vi "Test Get Item by ID.vi"(8 "error in (no error)":errorcluster, 11 "Test Case In":refnum<class "Debugger Test.lvclass">) -> (0 "error out":errorcluster, 3 "Test Case Out":refnum<class "Debugger Test.lvclass">)   [LabVIEW 2020, in "Debugger Test.lvclass"]
uses:
  Debugger Test.lvclass
  C:/Program Files (x86)/National Instruments/LabVIEW 2020/vi.lib/Astemes/LUnit/Test Case.lvclass
  source/Debugger/Debugger.lvclass
  C:/Users/anton/Documents/GitHub/triarc-debugger/source/Process/Debug Process.lvclass
  source/Debug Data/Raw Debug Data.ctl
  source/Debug Data/Debug Data.lvclass/Debug Data.ctl
  source/Process/Debug Process.lvclass/Debug Process.ctl
  <vilib>/Astemes/LUnit/Test Case.lvclass/Test Case.ctl
  <vilib>/Astemes/LUnit/LUnit Assertion Result.lvclass/LUnit Assertion Result.ctl
  <vilib>/Astemes/LUnit/LUnit Test Case Result.lvclass/LUnit Test Case Result.ctl
  <vilib>/Astemes/LUnit/LUnit Method Result.lvclass/LUnit Method Result.ctl
  01074fa8-ee8a-411d-bc8b-fc92c4f90959.vi
  source/Process/Private/SubVIs/Wait for finish.vi
  source/Process/Protected/Messaging/Enqueue Message.vi
  source/Process/Private/SubVIs/Set Lifecycle State.vi
  source/Process/Public/Lifecycle/Get Lifecycle State.vi
  <vilib>/Astemes/LUnit/Palette/Pass.vi
  <vilib>/Astemes/LUnit/Palette/Fail.vi
  <vilib>/Astemes/LUnit/Compare Variants.vi
  <vilib>/Astemes/LUnit/Describe Comparison.vi
  <vilib>/Astemes/LUnit/Set Assertion Type.vi
  <vilib>/Utility/error.llb/Clear Errors.vi
  <vilib>/Astemes/LUnit/Add test result.vi
  <vilib>/Astemes/LUnit/LUnit Write Passed.vi
  <vilib>/Astemes/LUnit/LUnit Write Message.vi
  <vilib>/Astemes/LUnit/LUnit Write Description.vi
  <vilib>/Astemes/LUnit/Variant to string.vi
  <vilib>/Astemes/LUnit/LUnit Write Assertion Type.vi
  <vilib>/Astemes/LUnit/LUnit Record Assertion Result.vi
  <vilib>/Astemes/LUnit/LUnit Aggregate Assertion Results.vi
  <vilib>/Astemes/LUnit/Assertion Result/LUnit Read Status.vi
  <vilib>/Astemes/LUnit/LUnit Read Message.vi
  <vilib>/Astemes/LUnit/LUnit Read Description.vi
  <vilib>/Astemes/LUnit/Method Result/LUnit Merge Status.vi
  <vilib>/Astemes/LUnit/LUnit Concatenate result strings.vi
  <vilib>/Utility/error.llb/Error Cluster From Error Code.vi
  <vilib>/Utility/Data Type/Get Type Information.vi
  <vilib>/Utility/LVClass/Get LV Class Name.vi
  <vilib>/Astemes/LUnit/LUnit Assertion Result.lvclass
  source/Process/Debug Process.lvclass
  source/Debug Data/Debug Data.lvclass
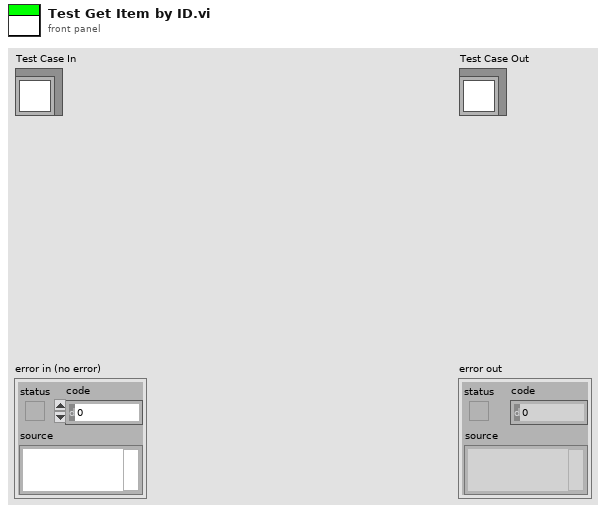
[diagram p1: front panel]
types:
  T1 = typedef "Debug Data.lvclass/Raw Debug Data.ctl" = cluster{"Action":string, "Call Chain":string, "Process":string, "Message":string, "Message Data":variant, "Time":dbl}
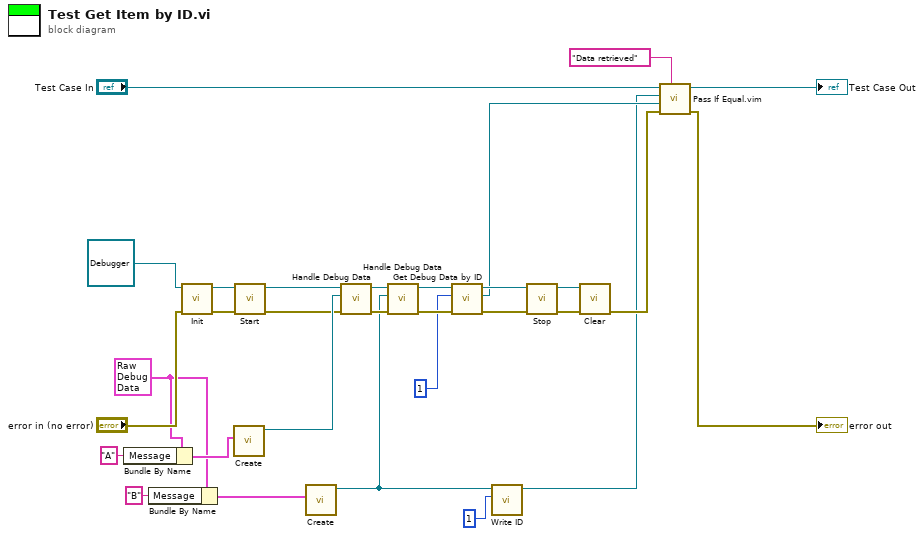
[diagram p0: block diagram]
diagram:
  w11 = T1 {"Action"="", "Call Chain"="", "Process"="", "Message"="", "Message Data"=variant, "Time"=0.0} ("Debug Data Cluster")
  n1 = Bundle By Name(cluster=w11, "Message"="A" ("Process")) -> (w18:T1)
  n2 = Bundle By Name(cluster=w11, "Message"="B" ("Process")) -> (w12:T1)
  n3 = call-dynamic "Init.vi"("error in (no error)"="error in (no error)", "Process In"=refnum<class "Debugger.lvclass"> refnum ("Debug Data Event In 2")) -> ("error out"=w26:errorcluster, "Process Out"=w27:refnum<class "Debugger.lvclass">)  [unwired: 8 in]
  n4 = call "Create.vi"("Debug Data Cluster"=w18) -> ("Debug Data out"=w19:refnum<class "Debug Data.lvclass">)  [unwired: 9 in, 1 out]
  n5 = call "Start.vi"("error in (no error)"=w26, "Process In"=w27) -> ("error out"=w4:errorcluster, "Process Out"=w5:refnum<class "Debugger.lvclass">)  [unwired: 7 in, 1 out]
  n6 = call "Create.vi"("Debug Data Cluster"=w12) -> ("Debug Data out"=w6:refnum<class "Debug Data.lvclass">)  [unwired: 9 in, 1 out]
  n7 = call-dynamic "Handle Debug Data.vi"("error in (no error)"=w4, "Debug Data.lvclass"=w19, "Debug Data Event In"=w5) -> ("error out"=w15:errorcluster, "Debug Data Event Out"=w16:refnum<class "Debugger.lvclass">)  [unwired: 7 in]
  n8 = call-dynamic "Handle Debug Data.vi"("error in (no error)"=w15, "Debug Data.lvclass"=w6, "Debug Data Event In"=w16) -> ("error out"=w14:errorcluster, "Debug Data Event Out"=w9:refnum<class "Debugger.lvclass">)  [unwired: 7 in]
  n9 = call "Get Debug Data by ID.vi"("error in (no error)"=w14, "Message ID"=u32 1, "Debugger In"=w9) -> ("error out"=w10:errorcluster, "Debug Data"=w3:refnum<class "Debug Data.lvclass">, "Debugger Out"=w8:refnum<class "Debugger.lvclass">)  [unwired: 6 in]
  n10 = call "Write ID.vi"("ID"=u32 1 ("Message ID"), "Debug Data in"=w6) -> ("Debug Data out"=w2:refnum<class "Debug Data.lvclass">)  [unwired: 8 in, 1 out]
  n11 = call "Stop.vi"("error in (no error)"=w10, "Process In"=w8) -> ("error out"=w24:errorcluster, "Process Out"=w25:refnum<class "Debugger.lvclass">)  [unwired: 7 in, 1 out]
  n12 = call-dynamic "Clear.vi"("error in (no error)"=w24, "Process In"=w25) -> ("error out"=w21:errorcluster)  [unwired: 9 in]
  n13 = call "Pass If Equal.vim"("Description"="Data retrieved", "error in (no error)"=w21, "Actual"=w3, "Expected"=w2, "LUnit Test Case In"="Test Case In") -> ("error out"=→"error out":errorcluster, "LUnit Test Case Out"=→"Test Case Out":refnum<class "Debugger Test.lvclass">)  [unwired: 5 in]
